vi "Read ini Error.vi"(9 "Error Code":string, 11 "Error Code file path":path) -> (3 "Error message":string[](array[string]))   [LabVIEW 2015]
uses:
  <vilib>/Utility/config.llb/Read Key (String).vi
  <vilib>/Utility/config.llb/NI_LVConfig.lvlib
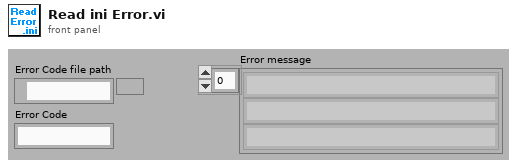
[diagram p1: front panel]
types:
  T1 = typedef "NI_LVConfig.lvlib/Config Data RefNum.ctl" = refnum<k1>
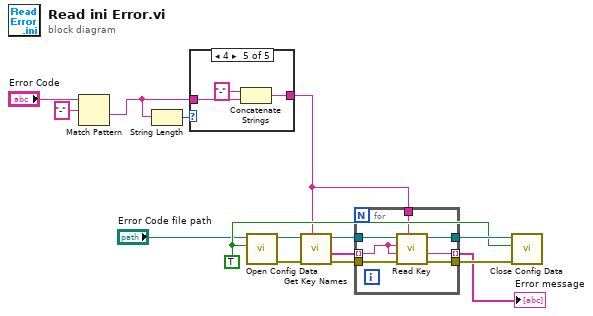
[diagram p0: block diagram]
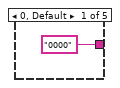
[diagram p2: hidden frame]
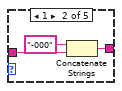
[diagram p3: hidden frame]
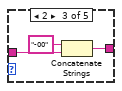
[diagram p4: hidden frame]
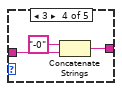
[diagram p5: hidden frame]
diagram:
  w8 = TRUE ("create file if necessary? (T)")
  n1 = Match Pattern(string="Error Code", regular expression="-") -> (after substring=w2:string)  [unwired: 1 in, 3 out]
  n2 = String Length(string=w2) -> (length=w5:i32)
  n3 = case shown="4" w5 {
    tunnel: w2 -> [_ w19 w21 w24 w27]
    tunnel: ["0000" ("¦r¦ê(I)") w17 w22 w25 w28] -> w4
    frame 0, Default {
    }
    frame 1 {
      n4 = Concatenate Strings("-000", w19) -> (w17:string)
    }
    frame 2 {
      n5 = Concatenate Strings("-00", w21) -> (w22:string)
    }
    frame 3 {
      n6 = Concatenate Strings("-0", w24) -> (w25:string)
    }
    frame 4 {
      n7 = Concatenate Strings("-", w27) -> (w28:string)
    }
  }
  n8 = call <vilib>:"Open Config Data.vi"("create file if necessary (T)"=w8, "configuration file path"="Error Code file path") -> ("error out"=w13:errorcluster, "refnum"=w15:T1)  [unwired: 7 in, 1 out]
  n9 = call <vilib>:"Get Key Names.vi"("section"=w4, "error in (no error)"=w13, "refnum"=w15) -> ("error out"=w12:errorcluster, "key names"=w11:string[], "refnum out"=w14:T1)  [unwired: 5 in, 1 out]
  n10 = for {
    tunnel: w14 -> [w35]
    tunnel: w12 -> [w34]
    tunnel: w4 -> [w33]
    tunnel: w11 -> [w32] mode=indexing
    tunnel: [w31] -> w6 mode=indexing
    tunnel: [w30] -> w10
    tunnel: [w29] -> w9
    n11 = call-poly <vilib>:"Read Key.vi"("section"=w33, "error in (no error)"=w34, "default value"=w32, "key"=w32, "refnum"=w35) -> ("error out"=w29:errorcluster, "value"=w31:string, "refnum out"=w30:T1)  [unwired: 3 in, 1 out]
  }
  "Error message" <- w6
  n12 = call <vilib>:"Close Config Data.vi"("error in (no error)"=w9, "write file if changed (T)"=w8, "refnum"=w10) -> ()  [unwired: 7 in, 2 out]
